vi "MetaClientPostProc.vi"(8 "error in (no error)":errorcluster, 11 "postproc action":enum16{"CONT_IDLE", "CONT_CONTIUE", "CONT_STOP"}(ring)) -> (0 "error out":errorcluster)   [LabVIEW 2019]
panel:
  out "what to do":string
  out "json from server":string
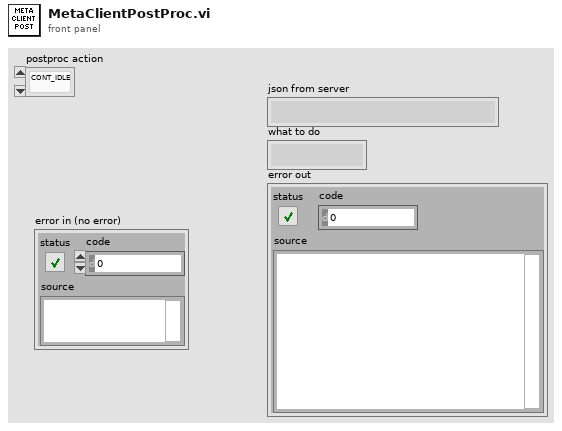
[diagram p1: front panel]
types:
  T1 = enum16{"Standard", "Buffered", "CRLF", "Immediate"}
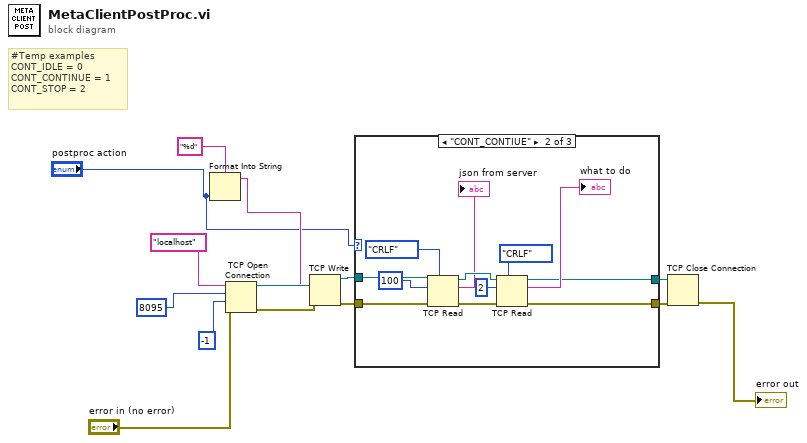
[diagram p0: block diagram]
diagram:
  # "#Temp examples\nCONT_IDLE = 0\nCONT_CONTINUE = 1\nCONT_STOP = 2"
  n1 = Format Into String(format string="%d", "postproc action") -> (resulting string=w2:string)  [unwired: 2 in, 1 out]
  n2 = TCP Open Connection(address="localhost", remote port or service name=u16 8095, timeout ms (60000)=-1, error in (no error)="error in (no error)") -> (connection ID=w11:refnum<k5>, error out=w10:errorcluster)  [unwired: 1 in]
  n3 = TCP Write(connection ID=w11, data in=w2, error in (no error)=w10) -> (connection ID out=w8:refnum<k5>, error out=w9:errorcluster)  [unwired: 1 in, 1 out]
  n4 = case shown="\"CONT_CONTIUE\"" "postproc action" {
    tunnel: w9 -> [w15 w28 w29]
    tunnel: w8 -> [w16 w27 w30]
    tunnel: [w15 w18 w29] -> w7
    tunnel: [w16 w17 w30] -> w6
    frame "CONT_IDLE", Default {
    }
    frame "CONT_CONTIUE" {
      n5 = TCP Read(connection ID=w27, bytes to read=100, error in (no error)=w28, 7:T1."CRLF" ("mode (standard)")) -> (connection ID out=w22:refnum<k5>, data out=→"json from server":string, error out=w24:errorcluster)  [unwired: 1 in]
      n6 = TCP Read(connection ID=w22, bytes to read=2, error in (no error)=w24, 7:T1."CRLF" ("mode (standard)")) -> (connection ID out=w17:refnum<k5>, data out=→"what to do":string, error out=w18:errorcluster)  [unwired: 1 in]
    }
    frame "CONT_STOP" {
    }
  }
  n7 = TCP Close Connection(connection ID=w6, error in (no error)=w7) -> (error out=→"error out":errorcluster)  [unwired: 1 in, 1 out]
